vi "二进制转10进制.vi"(1 "字符串":string) -> (0 "十进制数":i32)   [LabVIEW 2023]
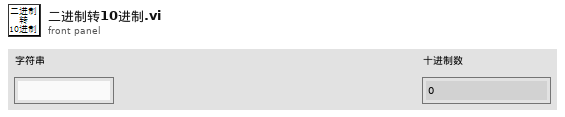
[diagram p1: front panel]
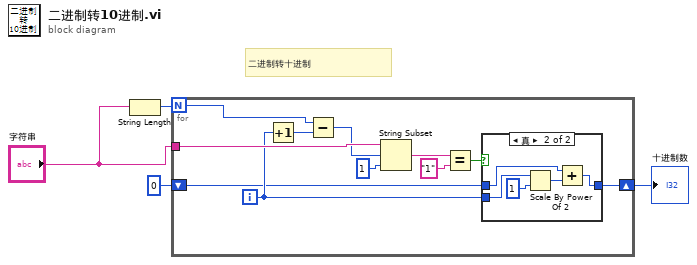
[diagram p0: block diagram]
diagram:
  # "二进制转十进制"
  n1 = String Length(string="字符串") -> (length=w4:i32)
  n2 = for {
    N: w4 -> [w13]
    tunnel: "字符串" -> [w15]
    shift-right: [w5] -> w2
    shift-left: 0 ("长度（剩余）") -> [w6]
    i -> [w7]
    n3 = Increment(x=w7) -> (x+1=w11:i32)
    n4 = Subtract(x=w13, y=w11) -> (x-y=w12:i32)
    n5 = String Subset(string=w15, offset (0)=w12, length (rest)=1 ("长度（剩余）")) -> (substring=w10:string)
    n6 = Equal?(x=w10, y="1") -> (x = y?=w8:bool)
    n7 = case shown="真" w8 {
      tunnel: w7 -> [_ w21]
      tunnel: w6 -> [w16 w20]
      tunnel: [w16 w18] -> w5
      frame False {
      }
      frame True {
        n8 = Scale By Power Of 2(n=w21, x=1) -> (x*2^n=w17:i32)
        n9 = Add(x=w20, y=w17) -> (x+y=w18:i32)
      }
    }
  }
  "十进制数" <- w2
